vi "LVClass_HasoSlopes Apply Scaler.vi"(0 "HasoSlopes in":refnum<class "HasoSlopes.lvclass">, 7 "Scaler":sgl, 11 "error in (no error)":errorcluster) -> (4 "HasoSlopes out":refnum<class "HasoSlopes.lvclass">, 15 "error out":errorcluster)   [LabVIEW 2020, in "HasoSlopes.lvclass"]
uses:
  HasoSlopes.lvclass
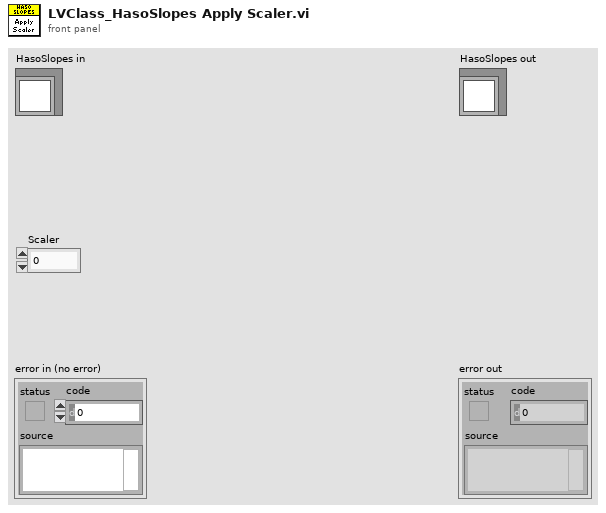
[diagram p1: front panel]
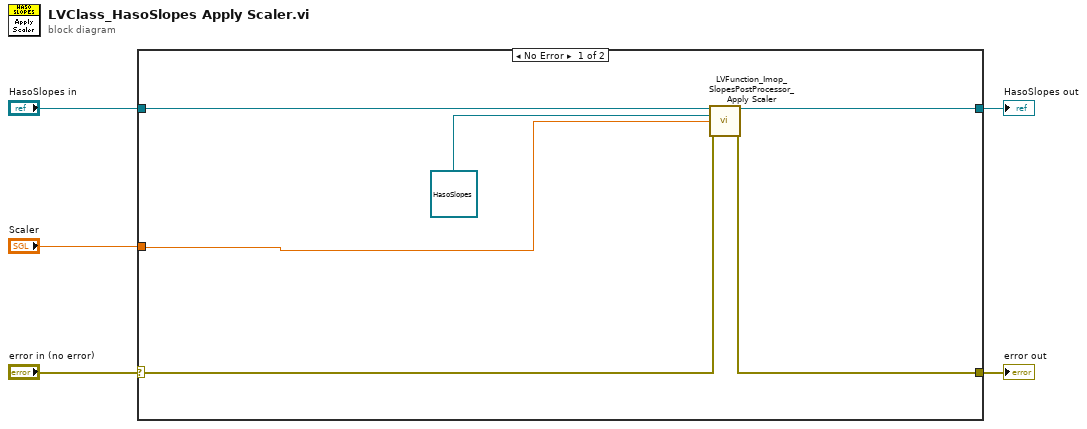
[diagram p0: block diagram]
diagram:
  n1 = case shown="No Error" "error in (no error)" {
    selector: "error in (no error)" -> [w10 w13]
    tunnel: [w9 w13] -> w4
    tunnel: [w7 w12] -> w2
    tunnel: "HasoSlopes in" -> [w11 w12]
    tunnel: "Scaler" -> [w8 _]
    frame No Error {
      n2 = call "LVFunction_Imop_SlopesPostProcessor_Apply Scaler.vi"("HasoSlopes in"=w11, "HasoSlopes OUT"=refnum<class "HasoSlopes.lvclass"> refnum, "Scaler"=w8, "error in (no error)"=w10) -> ("HasoSlopes out"=w7:refnum<class "HasoSlopes.lvclass">, "error out"=w9:errorcluster)  [unwired: 9 in, 1 out]
    }
    frame Error {
    }
  }
  "error out" <- w4
  "HasoSlopes out" <- w2
